vi "写入内置参数.vi"(7 "量程参数读取":T3 {"阈值（高->低）" format="%#.6g"; "阈值（低->高）" format="%#.6g"; "下限" format="%#.6g"; "上限" format="%#.6g"}, 8 "error in (no error)":errorcluster, 9 "float":T2 {"偏心轮校准参数" format="%#.6g"}, 10 "外设配置":T1 {"是否存在液位检测板" items=["否", "是"]; "阀数量" items=["9通"=9, "12通"=12]; "泵类型" items=["TECAN", "润泽"]}, 11 "MB session in":refnum<class "MB_Master.lvclass">) -> (0 "error out":errorcluster, 3 "MB session out":refnum<class "MB_Master.lvclass">)   [LabVIEW 2016, in "斯坦道CODMn新电路板.lvlib"]
uses:
  <vilib>/Plasmionique/MB Master/MB_Master/MB_Master.lvclass
  <vilib>/Plasmionique/MB Master/MB_Master_Serial/MB_Master_Serial.lvclass
  D:/Program Files (x86)/National Instruments/LabVIEW 2016/vi.lib/Plasmionique/MB Master/MB_Master/MB_Master.lvclass
  <vilib>/Plasmionique/MB Master/MB Master.lvlib
panel:
  in  "VISA Resource":refnum<visa-resource-name>
  in  "引用选择":enum16{"MB引用", "自建引用"}(ring)
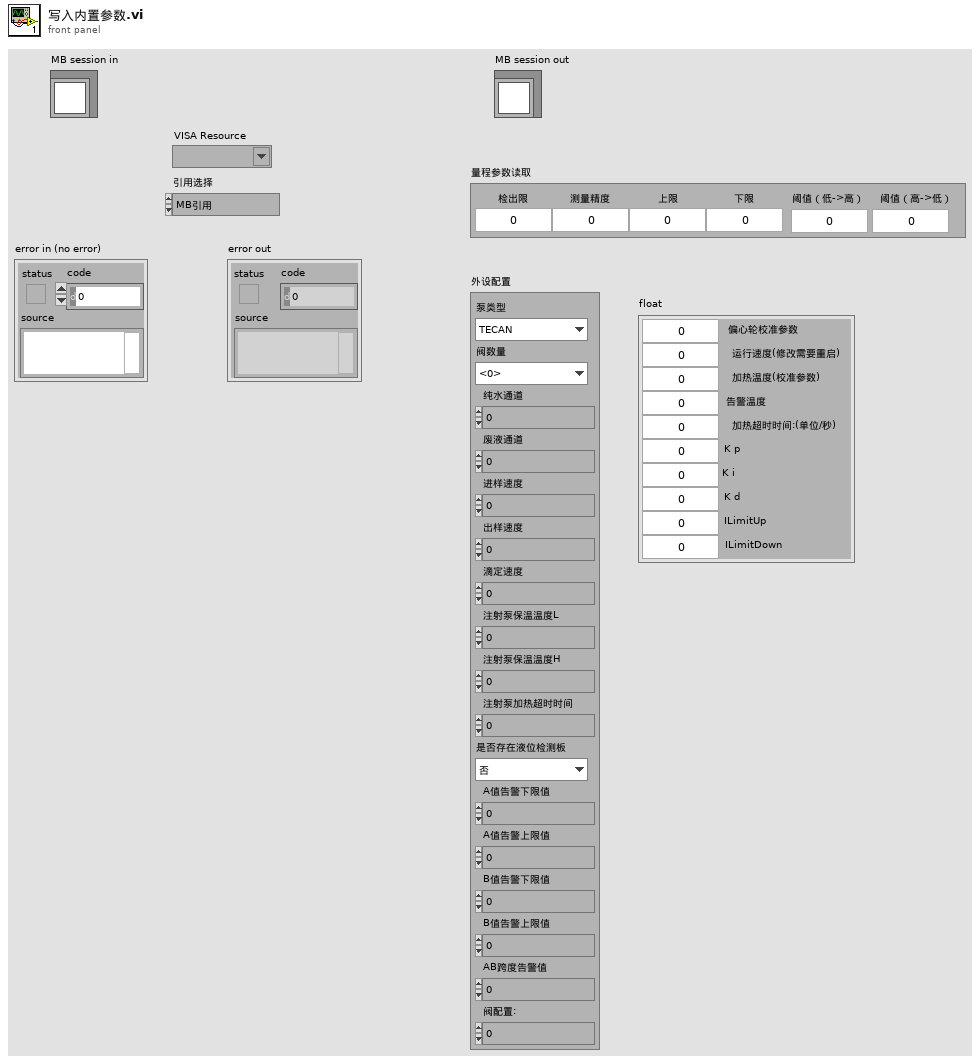
[diagram p1: front panel]
types:
  T1 = cluster{"泵类型":u8, "阀数量":u8, "纯水通道":u8, "废液通道":u8, "进样速度":u16, "出样速度":u16, "滴定速度":u16, "注射泵保温温度L":u8, "注射泵保温温度H":u8, "注射泵加热超时时间":u16, "是否存在液位检测板":u16, "A值告警下限值":u16, "A值告警上限值":u16, "B值告警下限值":u16, "B值告警上限值":u16, "AB跨度告警值":u16, "阀配置:":u8}
  T2 = cluster{"偏心轮校准参数":dbl, "运行速度(修改需要重启)":u16, "加热温度(校准参数) ":dbl, "告警温度":dbl, "加热超时时间:(单位/秒)":dbl, "K p":dbl, "K i":dbl, "K d":dbl, "ILimitUp":dbl, "ILimitDown":dbl}
  T3 = cluster{"检出限":dbl, "测量精度":dbl, "上限":dbl, "下限":dbl, "阈值（低->高）":dbl, "阈值（高->低）":dbl}
  T4 = cluster{"baud rate (bps)":u32, "stop bits":u16, "parity":u16, "flow control":u16, "timeout":u32, "retries":i32}
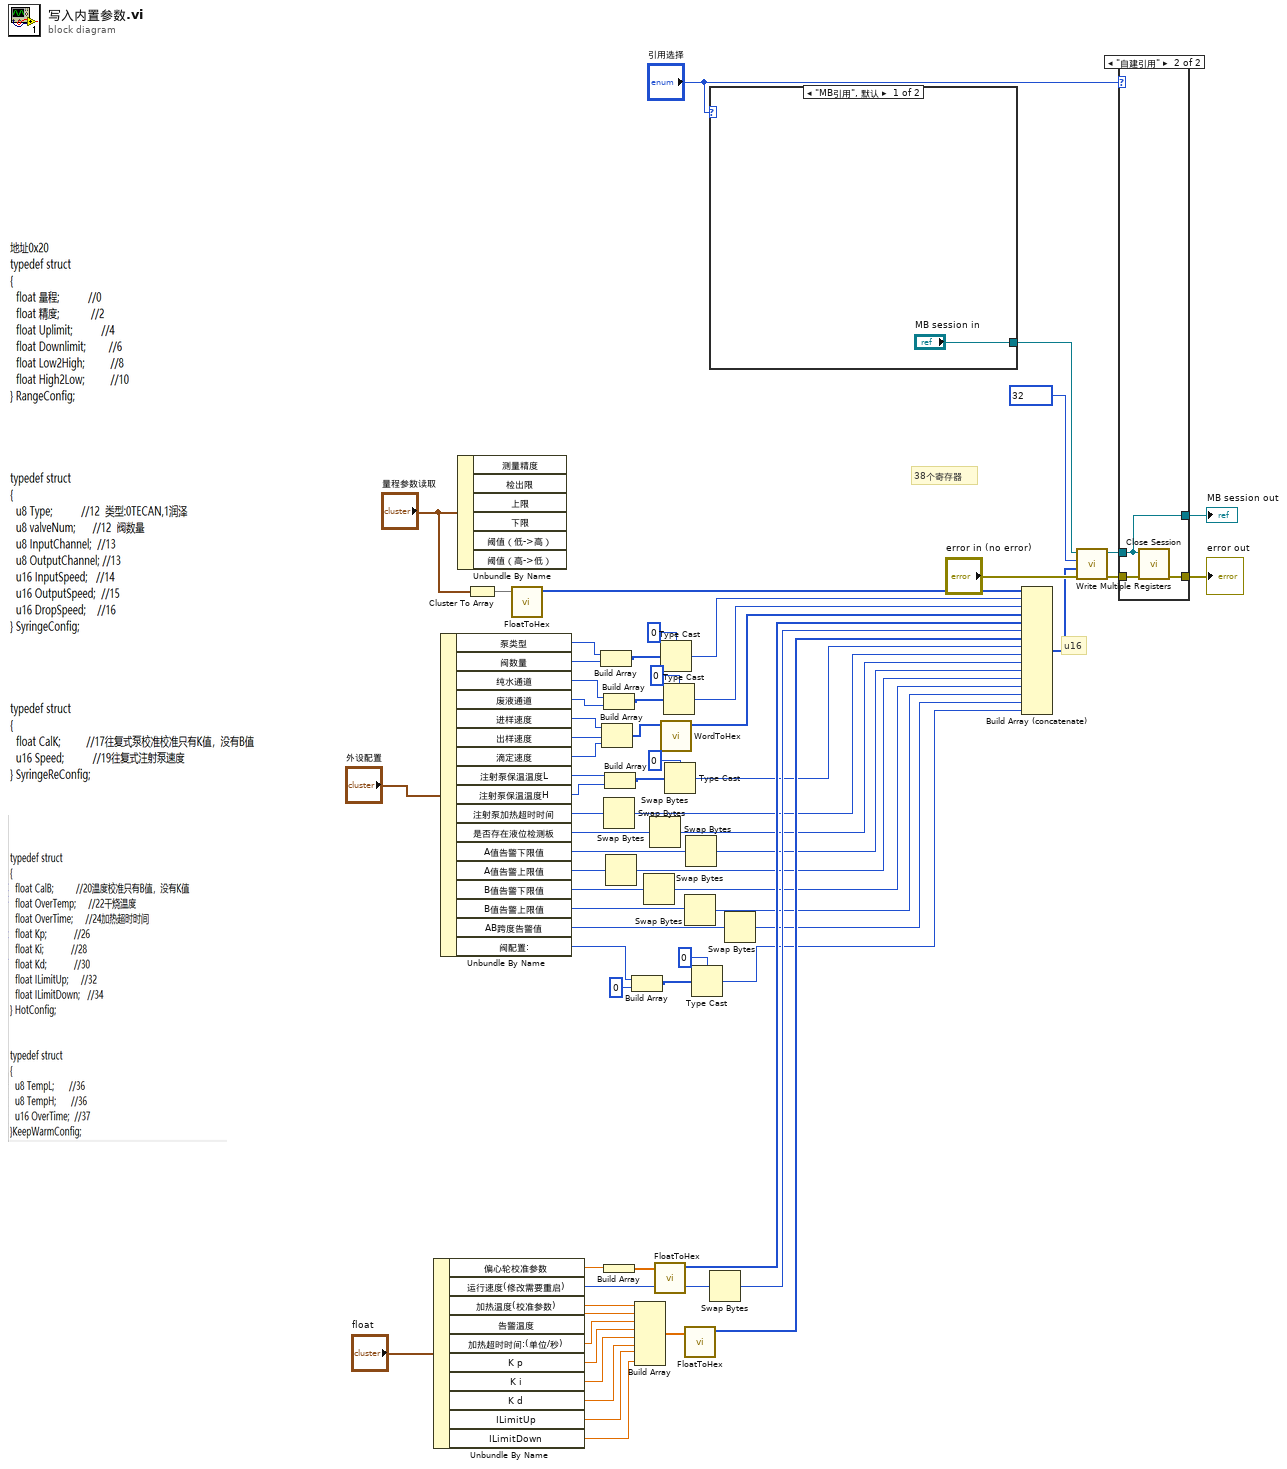
[diagram p0: block diagram]
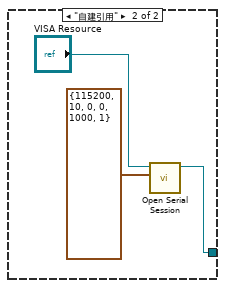
[diagram p3: hidden frame]
diagram:
  # "38个寄存器"
  # "u16"
  n1 = Unbundle By Name("float") -> ("偏心轮校准参数"=w45:dbl, "运行速度(修改需要重启)"=w22:u16, "加热温度(校准参数)"=w42:dbl, "告警温度"=w41:dbl, "加热超时时间:(单位/秒)"=w40:dbl, "K p"=w39:dbl, "K i"=w38:dbl, "K d"=w37:dbl, "ILimitUp"=w36:dbl, "ILimitDown"=w35:dbl)
  n2 = Unbundle By Name("外设配置") -> ("泵类型"=w57:u8, "阀数量"=w56:u8, "纯水通道"=w50:u8, "废液通道"=w49:u8, "进样速度"=w28:u16, "出样速度"=w27:u16, "滴定速度"=w26:u16, "注射泵保温温度L"=w31:u8, "注射泵保温温度H"=w30:u8, "注射泵加热超时时间"=w29:u16, "是否存在液位检测板"=w17:u16, "A值告警下限值"=w15:u16, "A值告警上限值"=w14:u16, "B值告警下限值"=w13:u16, "B值告警上限值"=w12:u16, "AB跨度告警值"=w11:u16, "阀配置:"=w3:u8)
  n3 = Unbundle By Name("量程参数读取") -> ()  [unwired: 6 out]
  n4 = Cluster To Array(cluster="量程参数读取") -> (array=w59:dbl[])
  n5 = call "FloatToHex.vi"("浮点数"=w59) -> ("DCBA整形输出"=w58:u16[])  [unwired: 10 in]
  n6 = Build Array(w57, w56) -> (w53:u8[])
  n7 = Build Array(w28, w27, w26) -> (w25:u16[])
  n8 = Build Array(w50, w49) -> (w52:u8[])
  n9 = Swap Bytes(anything=w29) -> (byte swapped=w18:u16)
  n10 = Build Array(w45) -> (w44:dbl[])
  n11 = Build Array(w31, w30) -> (w33:u8[])
  n12 = Swap Bytes(anything=w14) -> (byte swapped=w9:u16)
  n13 = Build Array(w3, u8 0 ("元素")) -> (w4:u8[])
  n14 = Build Array(w42, w41, w40, w39, w38, w37, w36, w35) -> (w34:dbl[])
  n15 = Swap Bytes(anything=w13) -> (byte swapped=w8:u16)
  n16 = Swap Bytes(anything=w17) -> (byte swapped=w16:u16)
  n17 = call "FloatToHex.vi"("浮点数"=w44) -> ("DCBA整形输出"=w23:u16[])  [unwired: 10 in]
  n18 = Type Cast(type=u16 0, x=w53) -> (*(type *) &x=w47:u16)
  n19 = call "WordToHex.vi"("WORD"=w25) -> ("数组"=w24:u16[])  [unwired: 10 in]
  n20 = Type Cast(type=u16 0, x=w52) -> (*(type *) &x=w46:u16)
  n21 = Type Cast(type=u16 0, x=w33) -> (*(type *) &x=w19:u16)
  n22 = Swap Bytes(anything=w12) -> (byte swapped=w7:u16)
  n23 = call "FloatToHex.vi"("浮点数"=w34) -> ("DCBA整形输出"=w20:u16[])  [unwired: 10 in]
  n24 = Swap Bytes(anything=w15) -> (byte swapped=w10:u16)
  n25 = Type Cast(type=u16 0, x=w4) -> (*(type *) &x=w2:u16)
  n26 = case shown="\"MB引用\", 默认" "引用选择" {
    tunnel: ["MB session in" w72] -> w66
    frame "MB引用", Default {
    }
    frame "自建引用" {
      n27 = call <vilib>:"Open Serial Session.vi"("Serial Config"=T4 {"baud rate (bps)"=115200, "stop bits"=10, "parity"=0, "flow control"=0, "timeout"=1000, "retries"=1}, "VISA Resource"="VISA Resource") -> ("MB_Serial session"=w72:refnum<class "MB_Master_Serial.lvclass">)  [unwired: 8 in, 1 out]
    }
  }
  n28 = Swap Bytes(anything=w22) -> (byte swapped=w21:u16)
  n29 = Swap Bytes(anything=w11) -> (byte swapped=w6:u16)
  n30 = Build Array (concatenate)(w58, w47, w46, w24, w23, w21, w20, w19, w18, w16, w10, w9, w8, w7, w6, w2) -> (w48:u16[])
  n31 = call <vilib>:"Write Multiple Registers.vi"("error in (no error)"="error in (no error)", "values"=w48, "starting address"=u16 32, "MB session in"=w66) -> ("error out"=w63:errorcluster, "MB session out"=w65:refnum<class "MB_Master.lvclass">)  [unwired: 6 in]
  n32 = case shown="\"自建引用\"" "引用选择" {
    tunnel: w65 -> [w73 w75]
    tunnel: w63 -> [w74 w77]
    tunnel: [w74 w76] -> w62
    tunnel: [w73 w75] -> w61
    frame "MB引用", Default {
    }
    frame "自建引用" {
      n33 = call-dynamic "Close Session.vi"("error in (no error)"=w77, "MB session in"=w75) -> ("error out"=w76:errorcluster)  [unwired: 9 in]
    }
  }
  "MB session out" <- w61
  "error out" <- w62
